vi "Adressen_F.vi"(13 "Aktion":T1) -> (4 "Messwerte":u16[](array[numeric]), 6 "Messbereich":u16[](array[numeric]), 8 "Kaliwerte":u16[](array[numeric]), 10 "Gerätestatus":u16[](array[numeric]))   [LabVIEW 2020, in "ABB-EL3000.lvlib" / "FID.lvlib"]
uses:
  FID.lvlib
  Aktion Adressen_F.ctl
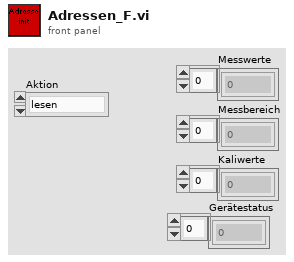
[diagram p1: front panel]
types:
  T1 = typedef "ABB-EL3000.lvlib/FID.lvlib/Aktion Adressen_F.ctl" = enum16{"lesen", "initialisieren"}
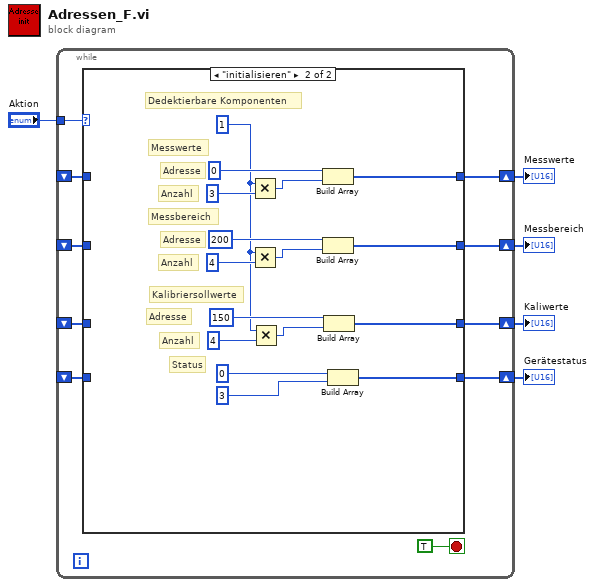
[diagram p0: block diagram]
diagram:
  n1 = while {
    shift-right: [w14] -> w4
    shift-left: _ -> [w13]
    tunnel: "Aktion" -> [w12]
    shift-right: [w11] -> w3
    shift-left: _ -> [w9]
    shift-right: [w10] -> w2
    shift-left: _ -> [w8]
    shift-right: [w7] -> w1
    shift-left: _ -> [w6]
    stop <- TRUE stop-if-true
    n2 = case shown="\"initialisieren\"" w12 {
      tunnel: [w19 w26] -> w14
      tunnel: w13 -> [w19 _]
      tunnel: [w18 w25] -> w11
      tunnel: [w17 w24] -> w10
      tunnel: w9 -> [w18 _]
      tunnel: w8 -> [w17 _]
      tunnel: [w16 w20] -> w7
      tunnel: w6 -> [w16 _]
      frame "lesen", Default {
      }
      frame "initialisieren" {
        w23 = u16 1
        # "Status"
        # "Anzahl"
        # "Adresse"
        # "Kalibriersollwerte"
        # "Anzahl"
        # "Adresse"
        # "Messbereich"
        # "Anzahl"
        # "Adresse"
        # "Messwerte"
        # "Dedektierbare Komponenten"
        n3 = Multiply(x=w23, y=u16 3) -> (x*y=w33:u16)
        n4 = Multiply(x=w23, y=u16 4) -> (x*y=w32:u16)
        n5 = Multiply(x=w23, y=u16 4) -> (x*y=w27:u16)
        n6 = Build Array(u16 0, w33) -> (w26:u16[])
        n7 = Build Array(u16 200, w32) -> (w25:u16[])
        n8 = Build Array(u16 150, w27) -> (w24:u16[])
        n9 = Build Array(u16 0, u16 3 ("Element")) -> (w20:u16[])
      }
    }
  }
  "Messwerte" <- w4
  "Messbereich" <- w3
  "Kaliwerte" <- w2
  "Gerätestatus" <- w1
